vi "Field_from_HP3478A.vi"(0 "GPIB Address":string="22") -> (1 "kOe":dbl, 2 "Tesla":dbl, 3 "Oe":dbl)   [LabVIEW 2015]
panel:
  out "Vout":dbl
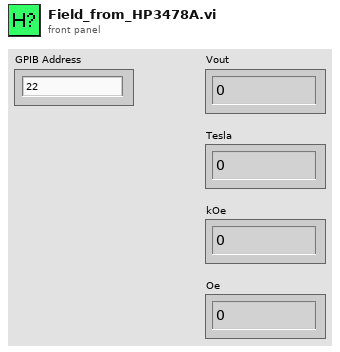
[diagram p1: front panel]
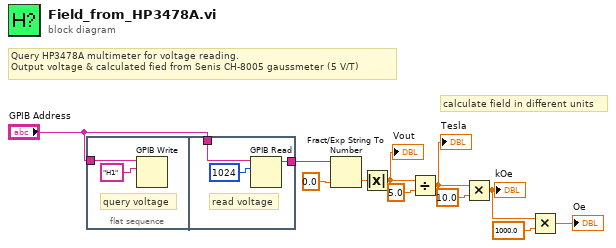
[diagram p0: block diagram]
diagram:
  # "calculate field in different units"
  # "Query HP3478A multimeter for voltage reading.\nOutput voltage & calculated fied from Senis CH-8005 gaussmeter (5 V/T)"
  n1 = flat-sequence {
    tunnel: "GPIB Address" -> [w12]
    tunnel: "GPIB Address" -> [w16]
    tunnel: [w14] -> w8
    frame #0 {
      # "query voltage"
      n2 = GPIB Write(0:w12, 1:"H1" ("data")) -> ()  [unwired: 3 in, 2 out]
    }
    frame #1 {
      # "read voltage"
      n3 = GPIB Read(0:w16, 1:1024 ("byte count")) -> (5:w14:string)  [unwired: 3 in, 2 out]
    }
  }
  n4 = Fract/Exp String To Number(string=w8, default (0 dbl)=0.0 ("default (0 I32)")) -> (number=w2:dbl)  [unwired: 2 in, 1 out]
  n5 = Absolute Value(x=w2) -> (abs(x)=w1:dbl)
  "Vout" <- w1
  n6 = Divide(x=w1, y=5.0) -> (x/y=w7:dbl)
  "Tesla" <- w7
  n7 = Multiply(x=w7, y=10.0) -> (x*y=w5:dbl)
  "kOe" <- w5
  n8 = Multiply(x=w5, y=1000.0) -> (x*y=→"Oe":dbl)
